vi "NoPieceCanMove.vi"(1 "LastMovePiece":cluster{"Row":i32, "Column":i32, "IsMove":bool}, 2 "Castling State":bool[][](array[boolean]), 3 "Black/White Turn (T/F)":bool, 4 "Board":i32[][](array[numeric])=[[-3, -5, -4, -2, -1, -4, -5, -3], [-6, -6, -6, -6, -6, -6, -6, -6], [0, 0, 0, 0, 0, 0, 0, 0], [0, 0, 0, 0, 0, 0, 0, 0], [0, 0, 0, 0, 0, 0, 0, 0], [0, 0, 0, 0, 0, 0, 0, 0], [6, 6, 6, 6, 6, 6, 6, 6], [3, 5, 4, 2, 1, 4, 5, 3]]) -> (0 "NoPieceCanMove":bool)   [LabVIEW 2014]
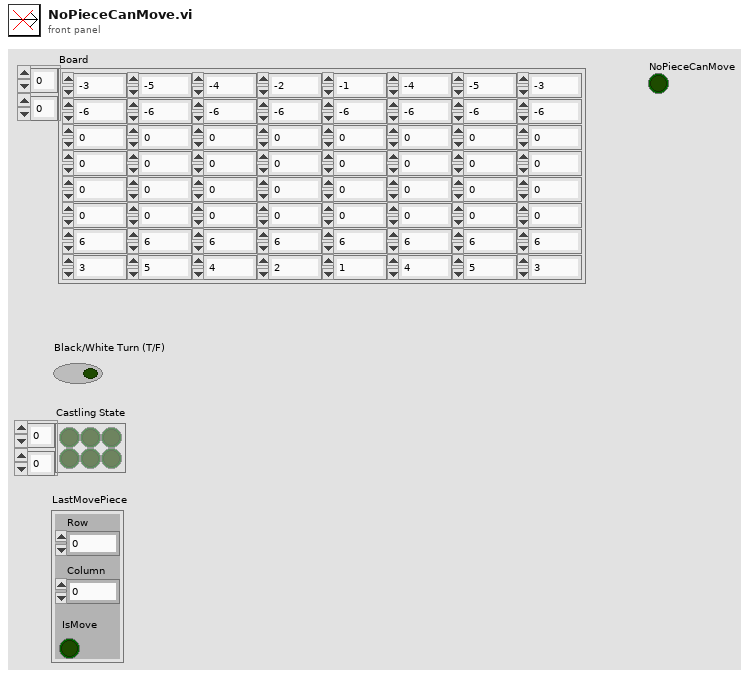
[diagram p1: front panel]
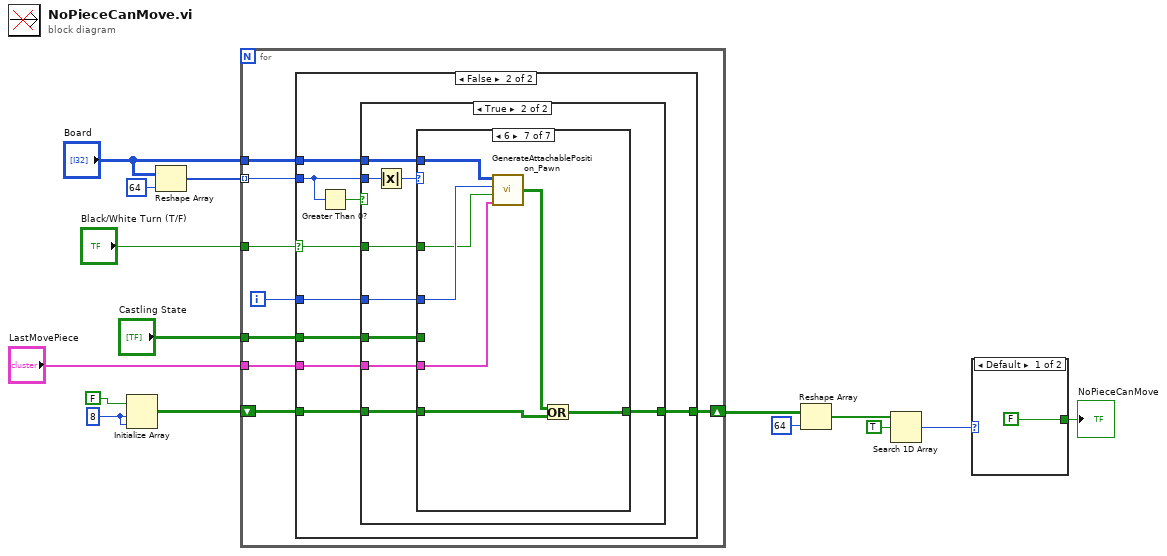
[diagram p0: block diagram]
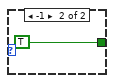
[diagram p2: hidden frame]
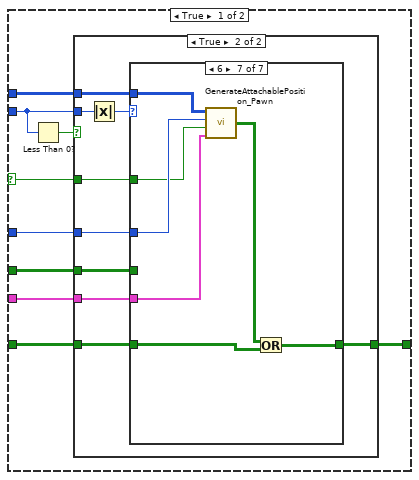
[diagram p3: hidden frame]
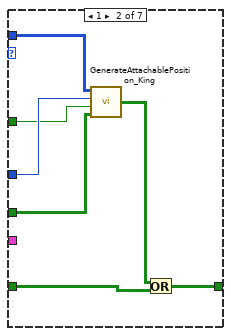
[diagram p6: hidden frame]
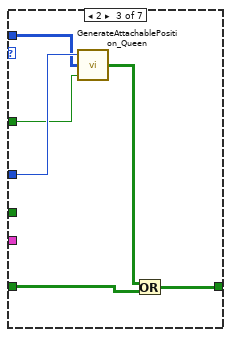
[diagram p7: hidden frame]
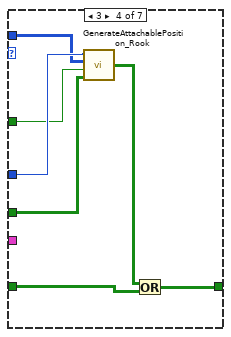
[diagram p8: hidden frame]
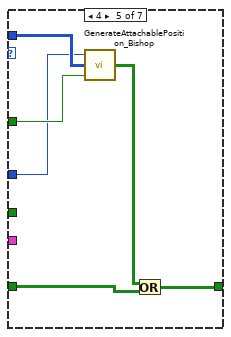
[diagram p9: hidden frame]
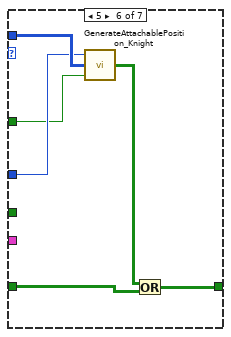
[diagram p10: hidden frame]
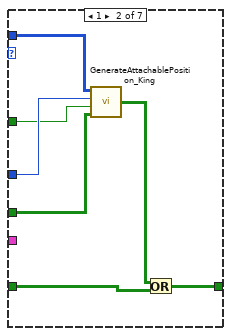
[diagram p13: hidden frame]
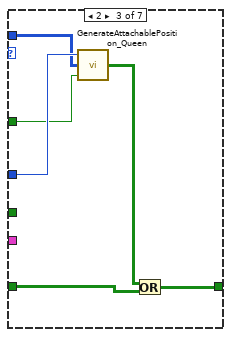
[diagram p14: hidden frame]
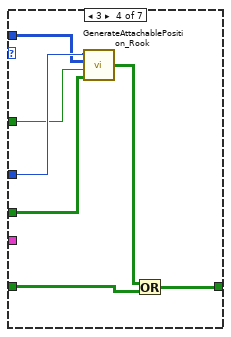
[diagram p15: hidden frame]
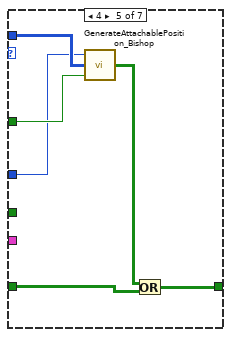
[diagram p16: hidden frame]
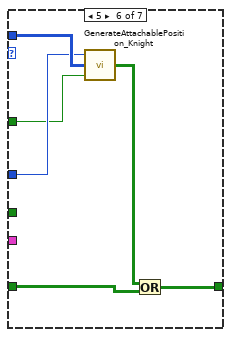
[diagram p17: hidden frame]
diagram:
  w15 = 8 ("dimension size")
  n1 = Initialize Array(FALSE, w15, w15) -> (w8:bool[][])
  n2 = Reshape Array("Board", 64 ("dimension size")) -> (w12:i32[])
  n3 = for {
    tunnel: w12 -> [w22] mode=indexing
    tunnel: "Black/White Turn (T/F)" -> [w23]
    tunnel: "Castling State" -> [w20]
    tunnel: "Board" -> [w19]
    shift-right: [w17] -> w6
    shift-left: w8 -> [w18]
    tunnel: "LastMovePiece" -> [w16]
    i -> [w21]
    n4 = case shown="False" w23 {
      selector: w23 -> [w29 w88]
      tunnel: w22 -> [w31 w90]
      tunnel: w21 -> [w30 w89]
      tunnel: w20 -> [w28 w87]
      tunnel: w19 -> [w27 w86]
      tunnel: w18 -> [w26 w85]
      tunnel: [w25 w84] -> w17
      tunnel: w16 -> [w24 w83]
      frame True {
        n5 = Less Than 0?(x=w31) -> (x < 0?=w32:bool)
        n6 = case shown="True" w32 {
          tunnel: w31 -> [_ w42]
          tunnel: w30 -> [_ w40]
          tunnel: w29 -> [_ w39]
          tunnel: w28 -> [_ w38]
          tunnel: w27 -> [_ w37]
          tunnel: w26 -> [w33 w36]
          tunnel: [w33 w35] -> w25
          tunnel: w24 -> [_ w34]
          frame False {
          }
          frame True {
            n7 = Absolute Value(x=w42) -> (abs(x)=w41:i32)
            n8 = case shown="6" w41 {
              tunnel: w40 -> [_ w50 w56 w60 w64 w71 w78]
              tunnel: w39 -> [_ w49 w54 w58 w66 w70 w77]
              tunnel: w38 -> [_ w48 _ w57 _ _ _]
              tunnel: w37 -> [_ w47 w55 w59 w65 w72 w79]
              tunnel: [w43 w46 w53 w63 w69 w75 w82] -> w35
              tunnel: w36 -> [w43 w45 w52 w62 w68 w74 w81]
              tunnel: w34 -> [_ _ _ _ _ _ w76]
              frame 0, Default {
              }
              frame 1 {
                n9 = call "GenerateAttachablePosition_King.vi"("Castling State"=w48, "Black/White Turn (T/F)"=w49, "pieceIndex"=w50, "Board"=w47) -> ("AttachablePosition"=w44:bool[][])
                n10 = Or(x=w44, y=w45) -> (x .or. y?=w46:bool[][])
              }
              frame 2 {
                n11 = call "GenerateAttachablePosition_Queen.vi"("Black/White Turn (T/F)"=w54, "Board"=w55, "pieceIndex"=w56) -> ("AttachablePosition"=w51:bool[][])
                n12 = Or(x=w51, y=w52) -> (x .or. y?=w53:bool[][])
              }
              frame 3 {
                n13 = call "GenerateAttachablePosition_Rook.vi"("Castling State"=w57, "Black/White Turn (T/F)"=w58, "Board"=w59, "pieceIndex"=w60) -> ("AttachablePosition"=w61:bool[][])
                n14 = Or(x=w61, y=w62) -> (x .or. y?=w63:bool[][])
              }
              frame 4 {
                n15 = call "GenerateAttachablePosition_Bishop.vi"("Black/White Turn (T/F)"=w66, "Board"=w65, "pieceIndex"=w64) -> ("AttachablePosition"=w67:bool[][])
                n16 = Or(x=w67, y=w68) -> (x .or. y?=w69:bool[][])
              }
              frame 5 {
                n17 = call "GenerateAttachablePosition_Knight.vi"("Black/White Turn (T/F)"=w70, "Board"=w72, "pieceIndex"=w71) -> ("AttachablePosition"=w73:bool[][])
                n18 = Or(x=w73, y=w74) -> (x .or. y?=w75:bool[][])
              }
              frame 6 {
                n19 = call "GenerateAttachablePosition_Pawn.vi"("LastMovePiece"=w76, "Black/White (T/F)"=w77, "pieceIndex"=w78, "Board"=w79) -> ("AttachablePosition"=w80:bool[][])
                n20 = Or(x=w80, y=w81) -> (x .or. y?=w82:bool[][])
              }
            }
          }
        }
      }
      frame False {
        n21 = Greater Than 0?(x=w90) -> (x > 0?=w91:bool)
        n22 = case shown="True" w91 {
          tunnel: w90 -> [_ w101]
          tunnel: w89 -> [_ w99]
          tunnel: w88 -> [_ w98]
          tunnel: w87 -> [_ w97]
          tunnel: w86 -> [_ w96]
          tunnel: w85 -> [w92 w95]
          tunnel: [w92 w94] -> w84
          tunnel: w83 -> [_ w93]
          frame False {
          }
          frame True {
            n23 = Absolute Value(x=w101) -> (abs(x)=w100:i32)
            n24 = case shown="6" w100 {
              tunnel: w99 -> [_ w109 w115 w119 w123 w130 w137]
              tunnel: w98 -> [_ w108 w113 w117 w125 w129 w136]
              tunnel: w97 -> [_ w107 _ w116 _ _ _]
              tunnel: w96 -> [_ w106 w114 w118 w124 w131 w138]
              tunnel: [w102 w105 w112 w122 w128 w134 w141] -> w94
              tunnel: w95 -> [w102 w104 w111 w121 w127 w133 w140]
              tunnel: w93 -> [_ _ _ _ _ _ w135]
              frame 0, Default {
              }
              frame 1 {
                n25 = call "GenerateAttachablePosition_King.vi"("Castling State"=w107, "Black/White Turn (T/F)"=w108, "pieceIndex"=w109, "Board"=w106) -> ("AttachablePosition"=w103:bool[][])
                n26 = Or(x=w103, y=w104) -> (x .or. y?=w105:bool[][])
              }
              frame 2 {
                n27 = call "GenerateAttachablePosition_Queen.vi"("Black/White Turn (T/F)"=w113, "Board"=w114, "pieceIndex"=w115) -> ("AttachablePosition"=w110:bool[][])
                n28 = Or(x=w110, y=w111) -> (x .or. y?=w112:bool[][])
              }
              frame 3 {
                n29 = call "GenerateAttachablePosition_Rook.vi"("Castling State"=w116, "Black/White Turn (T/F)"=w117, "Board"=w118, "pieceIndex"=w119) -> ("AttachablePosition"=w120:bool[][])
                n30 = Or(x=w120, y=w121) -> (x .or. y?=w122:bool[][])
              }
              frame 4 {
                n31 = call "GenerateAttachablePosition_Bishop.vi"("Black/White Turn (T/F)"=w125, "Board"=w124, "pieceIndex"=w123) -> ("AttachablePosition"=w126:bool[][])
                n32 = Or(x=w126, y=w127) -> (x .or. y?=w128:bool[][])
              }
              frame 5 {
                n33 = call "GenerateAttachablePosition_Knight.vi"("Black/White Turn (T/F)"=w129, "Board"=w131, "pieceIndex"=w130) -> ("AttachablePosition"=w132:bool[][])
                n34 = Or(x=w132, y=w133) -> (x .or. y?=w134:bool[][])
              }
              frame 6 {
                n35 = call "GenerateAttachablePosition_Pawn.vi"("LastMovePiece"=w135, "Black/White (T/F)"=w136, "pieceIndex"=w137, "Board"=w138) -> ("AttachablePosition"=w139:bool[][])
                n36 = Or(x=w139, y=w140) -> (x .or. y?=w141:bool[][])
              }
            }
          }
        }
      }
    }
  }
  n37 = Reshape Array(w6, 64 ("dimension size")) -> (w4:bool[])
  n38 = Search 1D Array(1D array=w4, element=TRUE) -> (index of element=w2:i32)  [unwired: 1 in]
  n39 = case shown="Default" w2 {
    tunnel: [FALSE TRUE] -> w1
    frame Default {
    }
    frame -1 {
    }
  }
  "NoPieceCanMove" <- w1
